vi "Read Python name.vi"(9 "PythonFunction in":refnum<class "PythonFunction.lvclass">) -> (3 "PythonFunction out":refnum<class "PythonFunction.lvclass">, 4 "Python name":string)   [LabVIEW 2014, in "PythonFunction.lvclass"]
uses:
  PythonFunction.lvclass
  PythonFunction.lvclass/PythonFunction.ctl
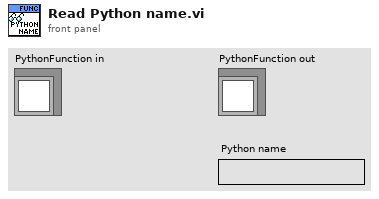
[diagram p1: front panel]
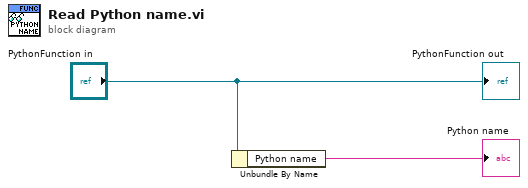
[diagram p0: block diagram]
diagram:
  n1 = Unbundle By Name("PythonFunction in") -> ("Python name"=→"Python name":string)
  "PythonFunction out" <- "PythonFunction in"
